vi "Zoom (BiLinear Interpolation).vi"(8 "error IN":errorcluster, 10 "Zoom Coefficient":dbl=1.0, 11 "image data IN":T1) -> (0 "error OUT":errorcluster, 3 "image data OUT":T1)   [LabVIEW 2026, in "image.lvlib"]
doc: "Created IvanLis by LabVIEW Portal\nProfile: http://labviewportal.org/memberlist.php?mode=viewprofile&u=987\neMail: IvanLisanov@gMail.com\nTelegram: https://t.me/IvanLis"
uses:
  image.lvlib
  <vilib>/picture/picture.llb/imagedata.ctl
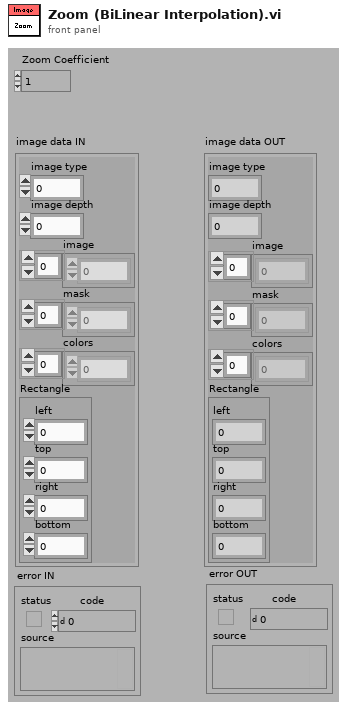
[diagram p1: front panel]
types:
  T1 = typedef "imagedata.ctl" = cluster{"image type":i32, "image depth":i32, "image":u8[], "mask":u8[], "colors":u32[], "Rectangle":cluster{"left":i16, "top":i16, "right":i16, "bottom":i16}}
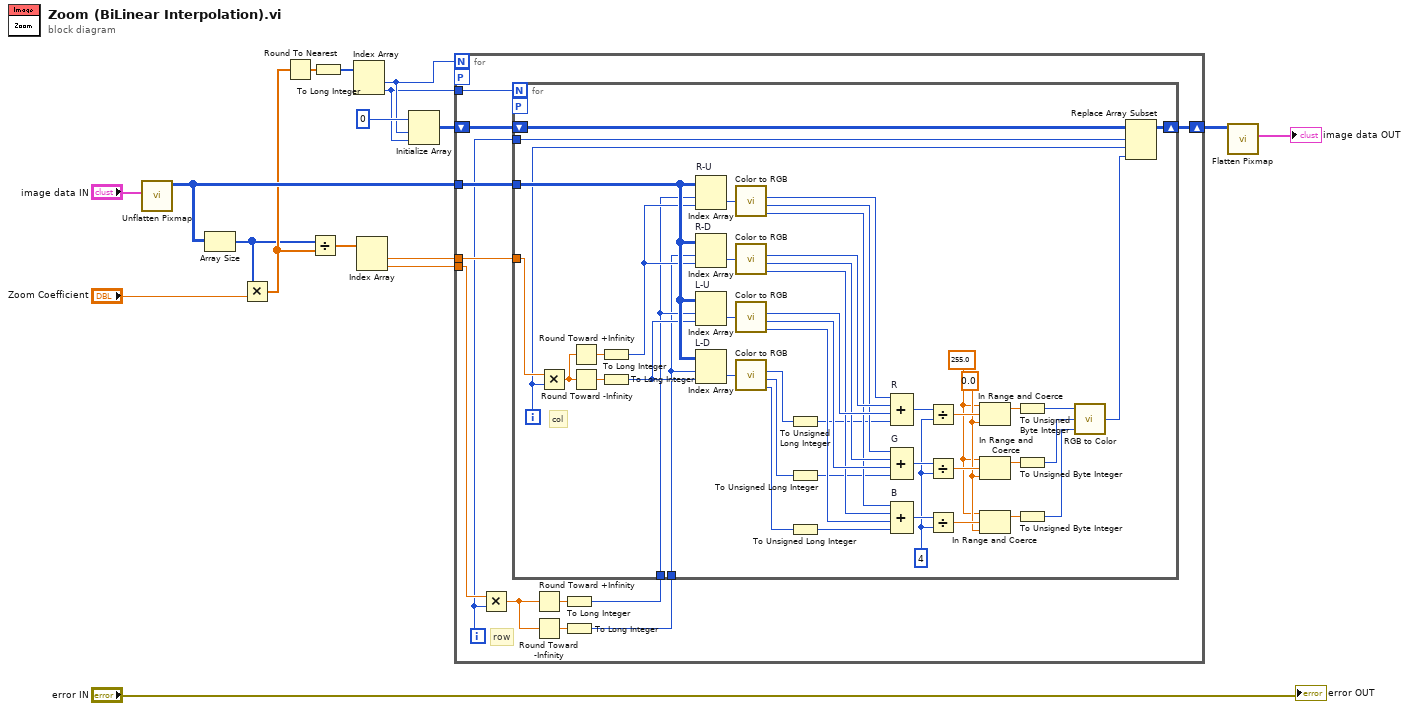
[diagram p0: block diagram]
diagram:
  n1 = call <vilib>:"Unflatten Pixmap.vi"("image data"="image data IN") -> ("24-bit pixmap"=w13:u32[][])  [unwired: 10 out]
  n2 = Array Size(array=w13) -> (size(s)=w7:i32[])
  n3 = Multiply(x=w7, y="Zoom Coefficient") -> (x*y=w9:dbl[])
  n4 = Round To Nearest(number=w9) -> (nearest integer value=w10:dbl[])
  n5 = Divide(x=w7, y=w9) -> (x/y=w12:dbl[])
  n6 = To Long Integer(number=w10) -> (32bit integer=w8:i32[])
  n7 = Index Array(array=w8) -> (element #1=w4:i32, element #2=w3:i32)  [unwired: 2 in]
  n8 = Index Array(array=w12) -> (element #1=w6:dbl, element #2=w11:dbl)  [unwired: 2 in]
  n9 = Initialize Array(u32 0 ("element"), w4, w3) -> (w2:u32[][])
  n10 = for {
    N: w4 -> [_]
    tunnel: w3 -> [w29]
    tunnel: w11 -> [w28]
    tunnel: w6 -> [w27]
    tunnel: w13 -> [w26]
    workers-P: _ -> [_]
    shift-right: [w19] -> w1
    shift-left: w2 -> [w20]
    i -> [w18]
    # "row"
    n11 = Multiply(x=w28, y=w18) -> (x*y=w22:dbl)
    n12 = Round Toward +Infinity(x=w22) -> (ceil(x): smallest int >= x=w24:dbl)
    n13 = Round Toward -Infinity(1:w22) -> (0:w23:dbl)
    n14 = To Long Integer(number=w24) -> (32bit integer=w21:i32)
    n15 = To Long Integer(number=w23) -> (32bit integer=w25:i32)
    n16 = for {
      N: w29 -> [_]
      tunnel: w27 -> [w77]
      tunnel: w26 -> [w73]
      tunnel: w25 -> [w49]
      tunnel: w21 -> [w50]
      workers-P: _ -> [_]
      shift-right: [w33] -> w19
      shift-left: w20 -> [w34]
      tunnel: w18 -> [w32]
      i -> [w31]
      w41 = 255.0 ("upper limit")
      w42 = 0.0 ("lower limit")
      w53 = 4
      # "col"
      n17 = Multiply(x=w77, y=w31) -> (x*y=w74:dbl)
      n18 = Round Toward +Infinity(x=w74) -> (ceil(x): smallest int >= x=w76:dbl)
      n19 = Round Toward -Infinity(1:w74) -> (0:w75:dbl)
      n20 = To Long Integer(number=w76) -> (32bit integer=w52:i32)
      n21 = To Long Integer(number=w75) -> (32bit integer=w51:i32)
      n22 = Index Array "R-U"(array=w73, index (row)=w50, index (col)=w52) -> (element=w69:u32)
      n23 = Index Array "R-D"(array=w73, index (row)=w49, index (col)=w52) -> (element=w72:u32)
      n24 = Index Array "L-U"(array=w73, index (row)=w50, index (col)=w51) -> (element=w71:u32)
      n25 = Index Array "L-D"(array=w73, index (row)=w49, index (col)=w51) -> (element=w70:u32)
      n26 = call <vilib>:"Color to RGB.vi"("Color"=w69) -> ("R"=w65:u8, "G"=w61:u8, "B"=w57:u8)  [unwired: 1 out]
      n27 = call <vilib>:"Color to RGB.vi"("Color"=w72) -> ("R"=w64:u8, "G"=w60:u8, "B"=w56:u8)  [unwired: 1 out]
      n28 = call <vilib>:"Color to RGB.vi"("Color"=w71) -> ("R"=w63:u8, "G"=w59:u8, "B"=w55:u8)  [unwired: 1 out]
      n29 = call <vilib>:"Color to RGB.vi"("Color"=w70) -> ("R"=w62:u8, "G"=w58:u8, "B"=w54:u8)  [unwired: 1 out]
      n30 = To Unsigned Long Integer(number=w62) -> (unsigned 32bit integer=w48:u32)
      n31 = To Unsigned Long Integer(number=w58) -> (unsigned 32bit integer=w47:u32)
      n32 = To Unsigned Long Integer(number=w54) -> (unsigned 32bit integer=w46:u32)
      n33 = Compound Arithmetic op=ADD "R"(w65, w64, w63, w48) -> (w68:u32)
      n34 = Compound Arithmetic op=ADD "G"(w61, w60, w59, w47) -> (w67:u32)
      n35 = Compound Arithmetic op=ADD "B"(w57, w56, w55, w46) -> (w66:u32)
      n36 = Divide(x=w68, y=w53) -> (x/y=w45:dbl)
      n37 = Divide(x=w67, y=w53) -> (x/y=w44:dbl)
      n38 = Divide(x=w66, y=w53) -> (x/y=w43:dbl)
      n39 = In Range and Coerce(upper limit=w41, x=w45, lower limit=w42) -> (coerced(x)=w37:dbl)  [unwired: 1 out]
      n40 = In Range and Coerce(upper limit=w41, x=w44, lower limit=w42) -> (coerced(x)=w36:dbl)  [unwired: 1 out]
      n41 = In Range and Coerce(upper limit=w41, x=w43, lower limit=w42) -> (coerced(x)=w35:dbl)  [unwired: 1 out]
      n42 = To Unsigned Byte Integer(number=w37) -> (unsigned 8bit integer=w39:u8)
      n43 = To Unsigned Byte Integer(number=w36) -> (unsigned 8bit integer=w40:u8)
      n44 = To Unsigned Byte Integer(number=w35) -> (unsigned 8bit integer=w38:u8)
      n45 = call <vilib>:"RGB to Color.vi"("B"=w38, "G"=w40, "R"=w39) -> ("Color"=w30:u32)
      n46 = Replace Array Subset(array=w34, new element=w30, index (row)=w32, index (col)=w31) -> (w33:u32[][])
    }
  }
  n47 = call <vilib>:"Flatten Pixmap.vi"("24-bit pixmap"=w1) -> ("image data"=→"image data OUT":T1)  [unwired: 6 in, 4 out]
  "error OUT" <- "error IN"
